vi "利用数列计算PI值1.vi"() -> (3 "PI":dbl format="%#_10g")   [LabVIEW 2012]
doc: "功能：\n\n利用数列求PI值。\n\n数列：\n\npi^2/4=1/1^2+1/2^2....+1/n^2.\n\nCSXCS_366创建"
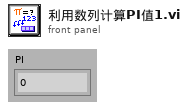
[diagram p1: front panel]
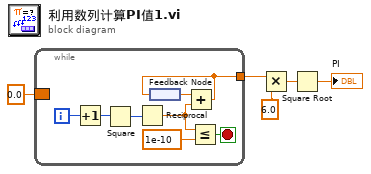
[diagram p0: block diagram]
diagram:
  n1 = while {
    tunnel: [w6] -> w3
    border: 0.0 -> [_]
    i -> [w11]
    stop <- w13 stop-if-true
    n2 = Increment(x=w11) -> (x+1=w10:i32)
    n3 = Square(x=w10) -> (x^2=w9:i32)
    n4 = Reciprocal(x=w9) -> (1/x=w8:dbl)
    n5 = feedback #1() -> (w7:dbl)
    n6 = Add(x=w7, y=w8) -> (x+y=w6:dbl)
    n7 = feedback-in #1(w6) -> ()
    n8 = Less Or Equal?(x=w8, y=1e-10) -> (x <= y?=w13:bool)
  }
  n9 = Multiply(x=w3, y=6.0) -> (x*y=w4:dbl)
  n10 = Square Root(x=w4) -> (sqrt(x)=→"PI":dbl)
